vi "pressure_set.vi"(8 "error in (no error)":errorcluster, 10 "Pressure in mbar":dbl, 11 "VISA resource name":refnum<visa-resource-name>) -> (0 "error out":errorcluster, 2 "Command string":string, 3 "VISA resource name out":refnum<visa-resource-name>)   [LabVIEW 2023]
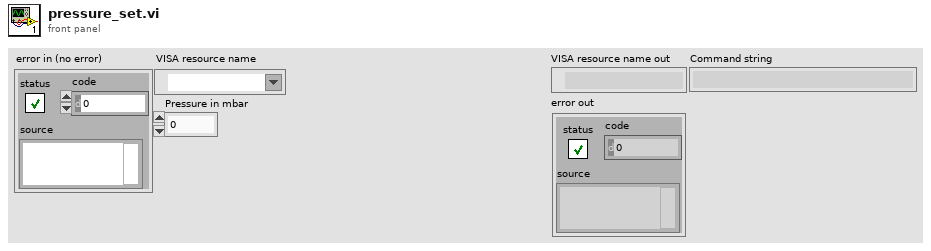
[diagram p1: front panel]
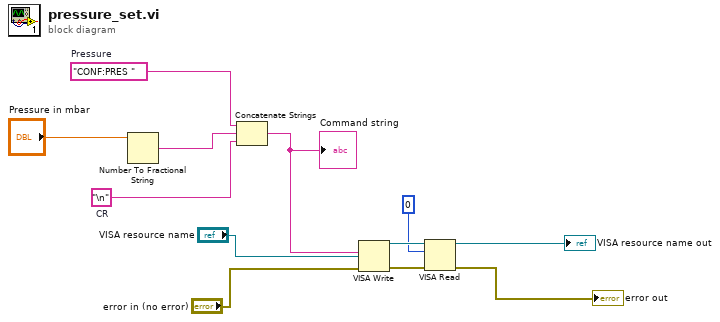
[diagram p0: block diagram]
diagram:
  w8 = "\n"  # CR
  w9 = "CONF:PRES "  # Pressure
  n1 = Number To Fractional String(number="Pressure in mbar") -> (F-format string=w10:string)  [unwired: 3 in]
  n2 = Concatenate Strings(w9, w10, w8) -> (w6:string)
  "Command string" <- w6
  n3 = VISA Write(VISA resource name="VISA resource name", write buffer=w6, error in (no error)="error in (no error)") -> (VISA resource name out=w5:refnum<visa-resource-name>, error out=w4:errorcluster)  [unwired: 1 out]
  n4 = VISA Read(VISA resource name=w5, byte count=u32 0, error in (no error)=w4) -> (VISA resource name out=→"VISA resource name out":refnum<visa-resource-name>, error out=→"error out":errorcluster)  [unwired: 2 out]
